vi "Open VISA Session Monitor.vi"() -> ()   [LabVIEW 2013]
panel:
  in  "Update every":sgl=0.5 min=0.1 step=0.1 format="%.1f"
  out "Number of \nOpen Sessions":i32
  in  "Quit":bool
  in  "Close":bool
  in  "Clear":bool
  in  "All":bool
  in  "Current Open Sessions":i32[](listbox)
  # "second(s)"
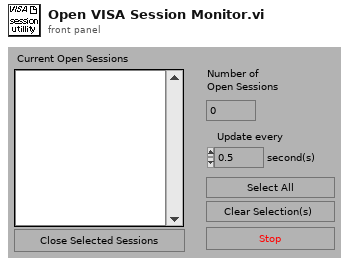
[diagram p1: front panel]
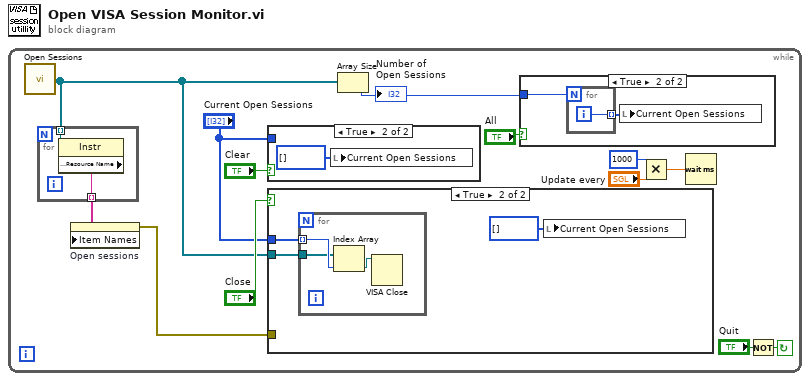
[diagram p0: block diagram]
diagram:
  n1 = while {
    stop <- w11 continue-if-true
    n2 = call <vilib>:"Open Sessions.vi"() -> ("Array of Refnums"=w2:refnum<visa-resource-name>[])  [unwired: 2 in]
    n3 = for {
      tunnel: w2 -> [w15] mode=indexing
      tunnel: [w14] -> w3 mode=indexing
      n4 = property class="Instr"(reference=w15) -> ("General Settings:Resource Name"=w14:string)  [unwired: 2 in, 1 out]
    }
    n5 = property on="Open sessions" class="LstBox (strict)"("Item Names"=w3) -> (error out=w1:errorcluster)  [unwired: 2 in, 1 out]
    n6 = case shown="True" "Clear" {
      tunnel: "Current Open Sessions" -> [_ _]
      frame False {
      }
      frame True {
        n7 = local write "Current Open Sessions"(i32[] [] ("Open sessions")) -> ()
      }
    }
    n8 = case shown="True" "Close" {
      tunnel: w2 -> [_ w21]
      tunnel: "Current Open Sessions" -> [_ w20]
      tunnel: w1 -> [_ _]
      frame False {
      }
      frame True {
        n9 = for {
          tunnel: w21 -> [w22]
          tunnel: w20 -> [w24] mode=indexing
          n10 = Index Array(array=w22, index=w24) -> (element=w23:refnum<visa-resource-name>)
          n11 = VISA Close(VISA resource name=w23) -> ()  [unwired: 1 in, 1 out]
        }
        n12 = local write "Current Open Sessions"(i32[] [] ("Open sessions")) -> ()
      }
    }
    n13 = Array Size(array=w2) -> (size(s)=w7:i32)
    "Number of \nOpen Sessions" <- w7
    n14 = case shown="True" "All" {
      tunnel: w7 -> [_ w16]
      frame False {
      }
      frame True {
        n15 = for {
          N: w16 -> [_]
          tunnel: [w18] -> w17 mode=indexing
          i -> [w18]
        }
        n16 = local write "Current Open Sessions"(w17) -> ()
      }
    }
    n17 = Multiply(x=u32 1000 ("milliseconds to wait"), y="Update every") -> (x*y=w4:sgl)
    n18 = Wait (ms)(milliseconds to wait=w4) -> ()  [unwired: 1 out]
    n19 = Not(x="Quit") -> (.not. x?=w11:bool)
  }
